vi "packetizer.vi"(10 "file path (use dialog)":path) -> (0 "ArtificialHorizon":picture, 1 "Heading Digital":dbl format="%.1f", 2 "Packet Payload":u8[](array[numeric]), 3 "CompassGauge":picture, 4 "Altitude  (/10000)":dbl, 5 "AltitudeIndicator":picture, 6 "VerticalSpeedDigital":dbl format="%.1f", 7 "VerticalSpeedIndicator":picture)   [LabVIEW 2023]
panel:
  in  "ScaleUnit(F=m; T=feet)":bool=TRUE
  out "count":u16
  out "MSG payload Len Arr":u8[](array[numeric])
  out "MSG Calc CRC":u16
  out "MSG CRC":u16
  out "MSG Payload":u8[](array[numeric])
  out "MSG Payload Len":u16
  out "MSG Class":u8
  out "MSG ID":u8
  in  "status":string="newpacket"
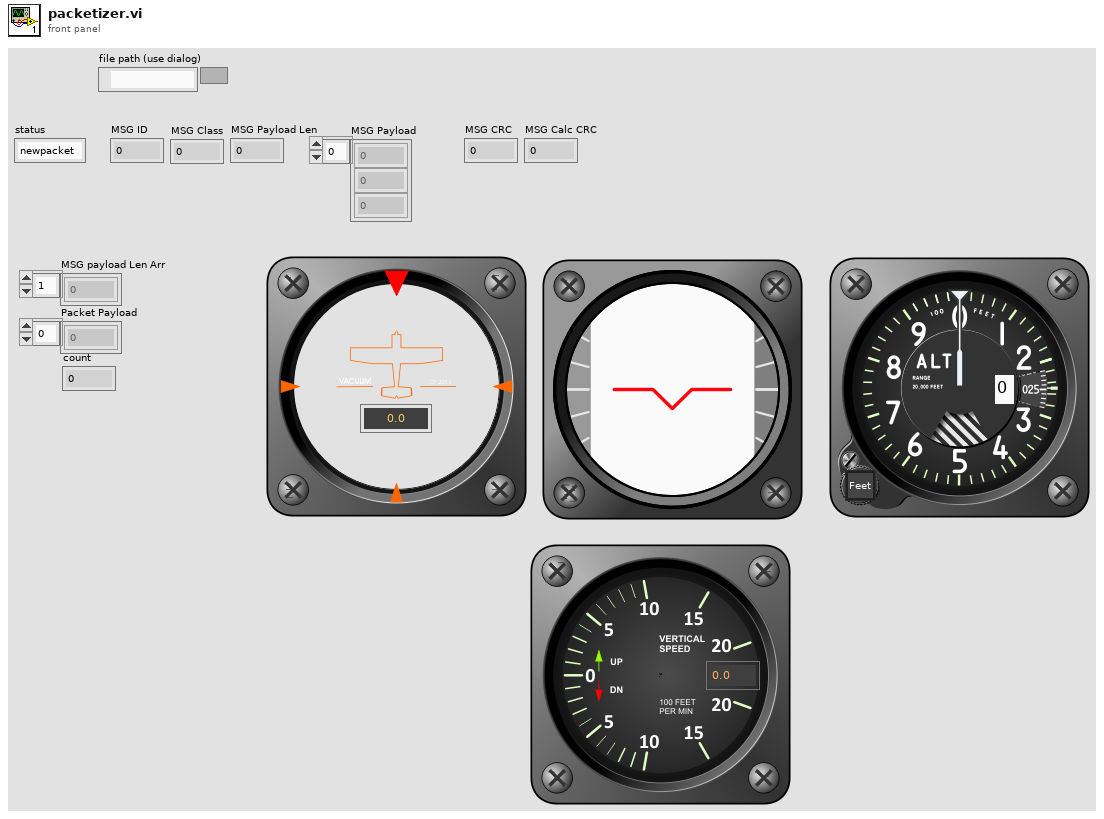
[diagram p1: front panel]
types:
  T1 = enum16{"big-endian, network order", "native, host order", "little-endian"}
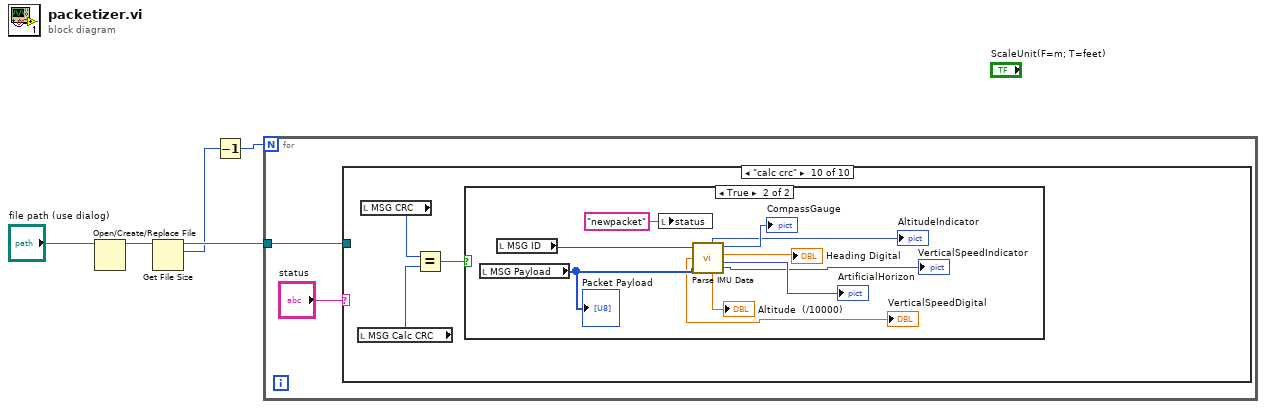
[diagram p0: block diagram]
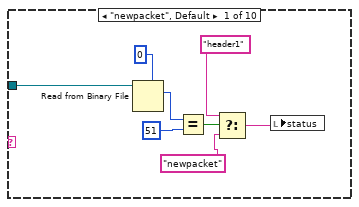
[diagram p2: hidden frame]
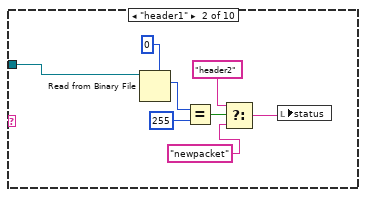
[diagram p3: hidden frame]
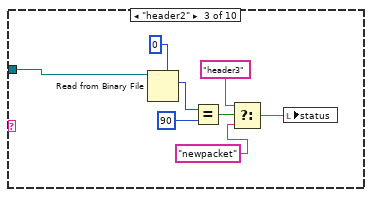
[diagram p4: hidden frame]
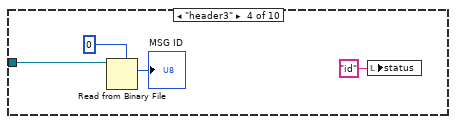
[diagram p5: hidden frame]
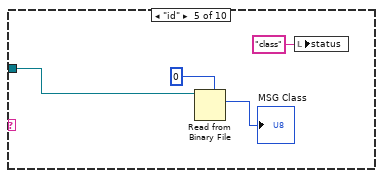
[diagram p6: hidden frame]
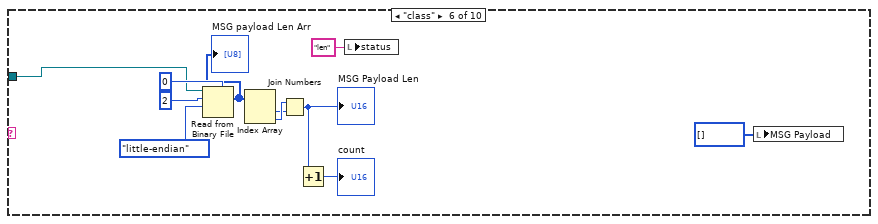
[diagram p7: hidden frame]
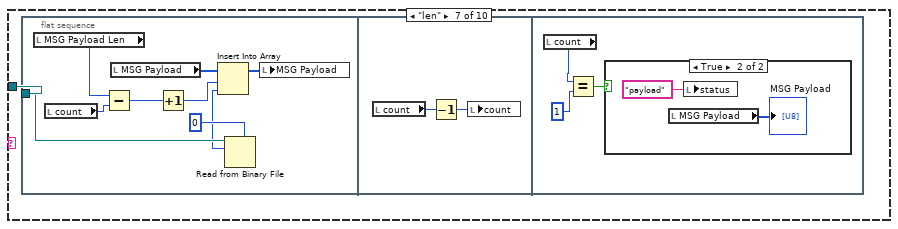
[diagram p8: hidden frame]
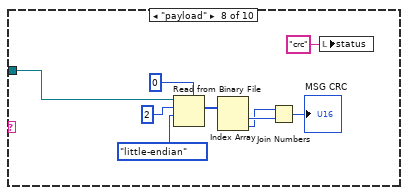
[diagram p10: hidden frame]
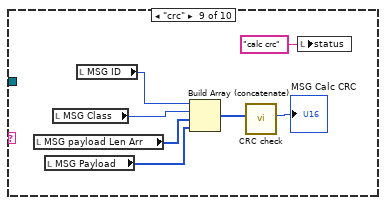
[diagram p11: hidden frame]
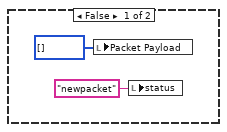
[diagram p12: hidden frame]
diagram:
  n1 = Open/Create/Replace File(file path (use dialog)="file path (use dialog)") -> (refnum out=w4:refnum<file>)  [unwired: 5 in, 2 out]
  n2 = Get File Size(file=w4) -> (refnum out=w3:refnum<file>, size (in bytes)=w2:i64)  [unwired: 1 in, 1 out]
  n3 = Decrement(x=w2) -> (x-1=w1:i64)
  n4 = for {
    N: w1 -> [_]
    tunnel: w3 -> [w6]
    n5 = case shown="\"calc crc\"" "status" {
      tunnel: w6 -> [w8 w16 w24 w32 w36 w43 w51 w68 _ _]
      frame "newpacket", Default {
        n6 = Read from Binary File(5:u8 0, 11:w8) -> (2:w13:u8)  [unwired: 4 in, 3 out]
        n7 = Equal?(x=w13, y=u8 51) -> (x = y?=w12:bool)
        n8 = Select(t="header1", s=w12, f="newpacket") -> (s? t:f=w9:string)
        n9 = local write "status"(w9) -> ()
      }
      frame "header1" {
        n10 = Read from Binary File(5:u8 0, 11:w16) -> (2:w21:u8)  [unwired: 4 in, 3 out]
        n11 = Equal?(x=w21, y=u8 255) -> (x = y?=w22:bool)
        n12 = Select(t="header2", s=w22, f="newpacket") -> (s? t:f=w23:string)
        n13 = local write "status"(w23) -> ()
      }
      frame "header2" {
        n14 = Read from Binary File(5:u8 0, 11:w24) -> (2:w30:u8)  [unwired: 4 in, 3 out]
        n15 = Equal?(x=w30, y=u8 90) -> (x = y?=w31:bool)
        n16 = Select(t="header3", s=w31, f="newpacket") -> (s? t:f=w25:string)
        n17 = local write "status"(w25) -> ()
      }
      frame "header3" {
        n18 = Read from Binary File(5:u8 0, 11:w32) -> (2:→"MSG ID":u8)  [unwired: 4 in, 3 out]
        n19 = local write "status"("id" ("status")) -> ()
      }
      frame "id" {
        n20 = Read from Binary File(5:u8 0, 11:w36) -> (2:→"MSG Class":u8)  [unwired: 4 in, 3 out]
        n21 = local write "status"("class" ("status")) -> ()
      }
      frame "class" {
        n22 = Read from Binary File(5:u8 0, 9:T1."little-endian" ("byte order (0:big-endian, network order)"), 10:2 ("count (1)"), 11:w43) -> (2:w44:u8[])  [unwired: 2 in, 3 out]
        "MSG payload Len Arr" <- w44
        n23 = Index Array(array=w44) -> (element #1=w47:u8, element #2=w48:u8)  [unwired: 2 in]
        n24 = Join Numbers(hi=w48, lo=w47) -> ((hi.lo)=w41:u16)
        "MSG Payload Len" <- w41
        n25 = Increment(x=w41) -> (x+1=→"count":u16)
        n26 = local write "status"("len" ("status")) -> ()
        n27 = local write "MSG Payload"(u8[] [] ("MSG Payload")) -> ()
      }
      frame "len" {
        n28 = flat-sequence {
          tunnel: w51 -> [w60]
          frame #0 {
            n29 = local read "MSG Payload Len"() -> (w57:u16)
            n30 = local read "count"() -> (w56:u16)
            n31 = Subtract(x=w57, y=w56) -> (x-y=w55:u16)
            n32 = local read "MSG Payload"() -> (w58:u8[])
            n33 = Increment(x=w55) -> (x+1=w54:u16)
            n34 = Read from Binary File(5:u8 0, 11:w60) -> (2:w53:u8)  [unwired: 4 in, 3 out]
            n35 = Insert Into Array(array=w58, index=w54, new element=w53) -> (w52:u8[])
            n36 = local write "MSG Payload"(w52) -> ()
          }
          frame #1 {
            n37 = local read "count"() -> (w62:u16)
            n38 = Decrement(x=w62) -> (x-1=w61:u16)
            n39 = local write "count"(w61) -> ()
          }
          frame #2 {
            n40 = local read "count"() -> (w65:u16)
            n41 = Equal?(x=w65, y=u16 1) -> (x = y?=w63:bool)
            n42 = case shown="True" w63 {
              frame False {
              }
              frame True {
                n43 = local read "MSG Payload"() -> (→"MSG Payload":u8[])
                n44 = local write "status"("payload" ("status")) -> ()
              }
            }
          }
        }
      }
      frame "payload" {
        n45 = Read from Binary File(5:u8 0, 9:T1."little-endian" ("byte order (0:big-endian, network order)"), 10:2 ("count (1)"), 11:w68) -> (2:w74:u8[])  [unwired: 2 in, 3 out]
        n46 = Index Array(array=w74) -> (element #1=w73:u8, element #2=w72:u8)  [unwired: 2 in]
        n47 = Join Numbers(hi=w72, lo=w73) -> ((hi.lo)=→"MSG CRC":u16)
        n48 = local write "status"("crc" ("status")) -> ()
      }
      frame "crc" {
        n49 = local read "MSG payload Len Arr"() -> (w80:u8[])
        n50 = local read "MSG Payload"() -> (w79:u8[])
        n51 = local read "MSG Class"() -> (w81:u8)
        n52 = local read "MSG ID"() -> (w82:u8)
        n53 = Build Array (concatenate)(w82, w81, w80, w79) -> (w78:u8[])
        n54 = call "CRC check.vi"("array"=w78) -> ("CRC"=→"MSG Calc CRC":u16)  [unwired: 10 in]
        n55 = local write "status"("calc crc" ("status")) -> ()
      }
      frame "calc crc" {
        n56 = local read "MSG Calc CRC"() -> (w85:u16)
        n57 = local read "MSG CRC"() -> (w86:u16)
        n58 = Equal?(x=w86, y=w85) -> (x = y?=w84:bool)
        n59 = case shown="True" w84 {
          frame False {
            n60 = local write "Packet Payload"(u8[] [] ("Packet Payload")) -> ()
            n61 = local write "status"("newpacket" ("status")) -> ()
          }
          frame True {
            n62 = local read "MSG Payload"() -> (w96:u8[])
            "Packet Payload" <- w96
            n63 = local read "MSG ID"() -> (w97:u8)
            n64 = local write "status"("newpacket" ("status")) -> ()
            n65 = call "Parse IMU Data.vi"("Packet"=w96, "ID"=w97) -> ("VerticalSpeedIndicator"=→"VerticalSpeedIndicator":picture, "Altitude  (/10000)"=→"Altitude  (/10000)":dbl, "ArtificialHorizon"=→"ArtificialHorizon":picture, "Heading Digital"=→"Heading Digital":dbl, "AltitudeIndicator"=→"AltitudeIndicator":picture, "CompassGauge"=→"CompassGauge":picture, "VerticalSpeedDigital"=→"VerticalSpeedDigital":dbl)
          }
        }
      }
    }
  }
